vi "CH COUPLING SETTING.vi"(8 "COUPLING:":enum32{"AC", "DC", "GND"}(radio), 10 "CHANNEL":enum32{"CH 1", "CH 2", "CH 3", "CH 4"}(radio), 11 "VISA resource name 2":refnum<visa-resource-name>="GPIB0::1::INSTR") -> ()   [LabVIEW 2018]
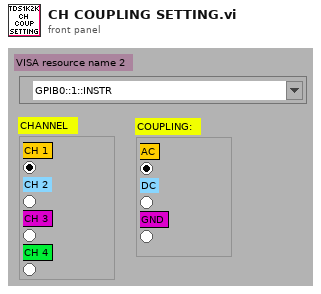
[diagram p1: front panel]
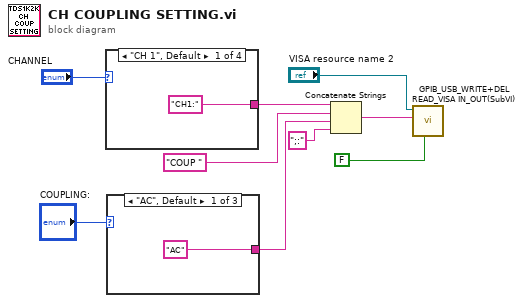
[diagram p0: block diagram]
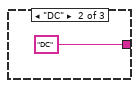
[diagram p2: hidden frame]
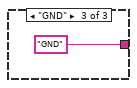
[diagram p3: hidden frame]
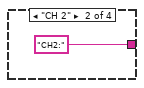
[diagram p4: hidden frame]
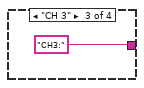
[diagram p5: hidden frame]
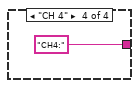
[diagram p6: hidden frame]
diagram:
  n1 = case shown="\"CH 1\", Default" "CHANNEL" {
    tunnel: ["CH1:" "CH2:" "CH3:" "CH4:"] -> w5
    frame "CH 1", Default {
    }
    frame "CH 2" {
    }
    frame "CH 3" {
    }
    frame "CH 4" {
    }
  }
  n2 = case shown="\"AC\", Default" "COUPLING:" {
    tunnel: ["AC" "DC" "GND"] -> w1
    frame "AC", Default {
    }
    frame "DC" {
    }
    frame "GND" {
    }
  }
  n3 = Concatenate Strings(w5, "COUP ", w1, ";:") -> (w8:string)
  n4 = call "GPIB_USB_WRITE+DEL READ_VISA IN_OUT(SubVI).vi"("VISA resource IN"="VISA resource name 2", "GPIB/USB WRITE"=w8, 4:FALSE ("READ GPIB")) -> ()  [unwired: 3 in, 3 out]
